vi "Centauro Verify LED Scroll.vi"(8 "Error In":errorcluster, 10 "#Retries":i32=20, 11 "GEA2 Reference In":refnum<k24>) -> (0 "Error Out":errorcluster, 2 "Pass/Fail?":bool, 3 "GEA2 Reference Out":refnum<k24>)   [LabVIEW 2016]
uses:
  Q:/Common/DLLs/GEA3/GeaCommunication.dll
  Common/DLLs/GEA3/GeaCommunication.dll
  Centauro Washer/Product Testcode/Centauro/Valew Common/type defs/LED Status OOB.ctl
  Common/LabVIEW GEA2 Toolkit/LabVIEW_GEA2_Toolkit.lvlibp
panel:
  in  "Board Index":i32
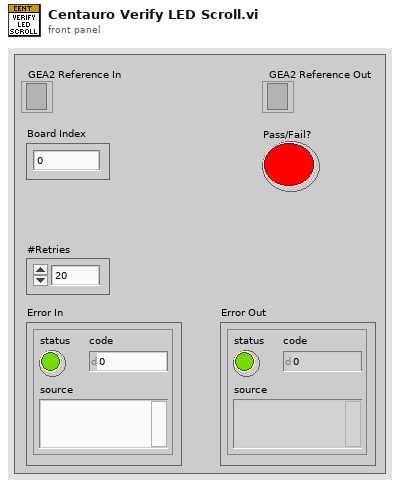
[diagram p1: front panel]
types:
  T1 = typedef "LED Status OOB.ctl" = enum32{"Off", "On", "Blink"}
  T2 = cluster{"Damp":T1, "Dry":T1, "Cool":T1, "Eco":T1}
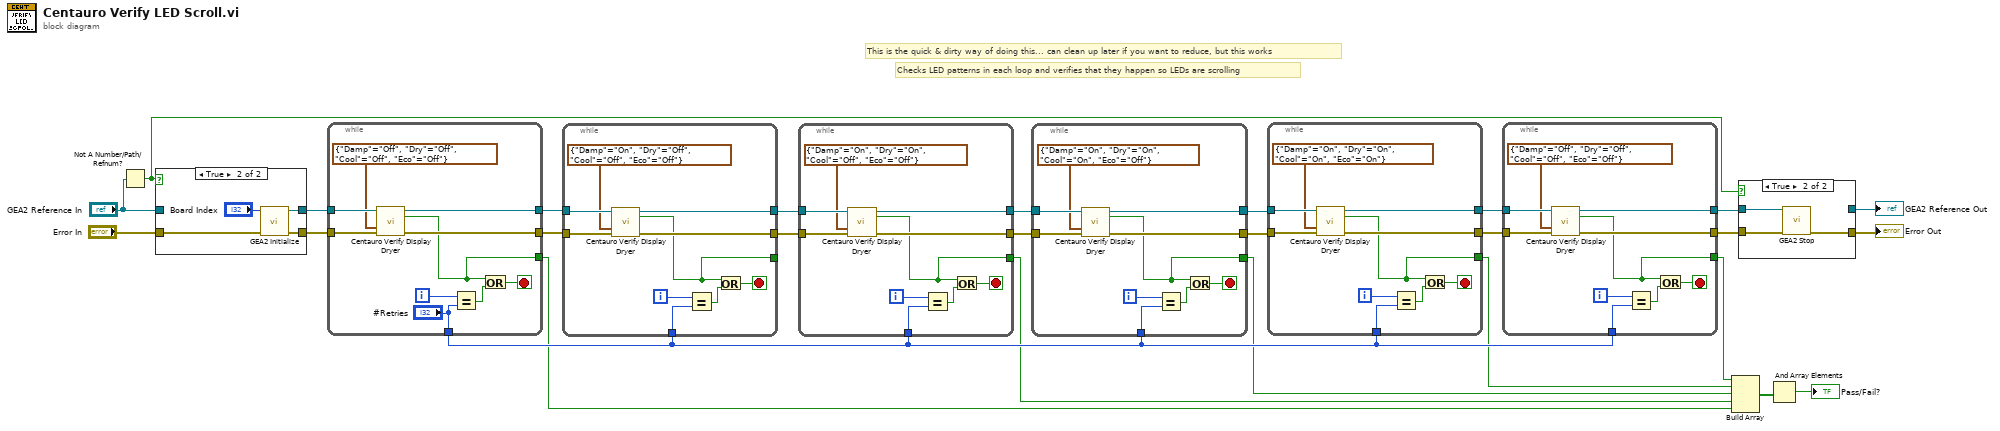
[diagram p0: block diagram]
diagram:
  # "Checks LED patterns in each loop and verifies that they happen so LEDs are scrolling"
  # "This is the quick & dirty way of doing this... can clean up later if you want to reduce, but this works"
  n1 = Not A Number/Path/Refnum?(number/path/refnum="GEA2 Reference In") -> (NaN/Path/Refnum?=w2:bool)
  n2 = case shown="True" w2 {
    tunnel: [w28 w33] -> w25
    tunnel: "Error In" -> [w28 w32]
    tunnel: [w29 w31] -> w26
    tunnel: "GEA2 Reference In" -> [w29 _]
    frame False {
    }
    frame True {
      n3 = call "GEA2 Initialize.vi"("Board Index"="Board Index", "error in"=w32) -> ("GEA2 Reference Out"=w31:refnum<k24>, "error out"=w33:errorcluster)  [unwired: 11 in, 1 out]
    }
  }
  n4 = while {
    tunnel: w26 -> [w43]
    tunnel: w25 -> [w42]
    tunnel: [w41] -> w24
    tunnel: [w40] -> w23
    tunnel: [w37] -> w9
    tunnel: ["#Retries"] -> w14
    i -> [w36]
    stop <- w38 stop-if-true
    n5 = call "Centauro Verify Display Dryer.vi"("GEA2 Reference In"=w43, "Expected LED Status"=T2 {"Damp"=enum."Off", "Dry"=enum."Off", "Cool"=enum."Off", "Eco"=enum."Off"}, "Error In"=w42) -> ("GEA2 Reference Out"=w41:refnum<k24>, "Pass/Fail?"=w37:bool, "Error Out"=w40:errorcluster)  [unwired: 7 in, 3 out]
    n6 = Equal?(x=w36, y="#Retries") -> (x = y?=w39:bool)
    n7 = Or(x=w37, y=w39) -> (x .or. y?=w38:bool)
  }
  n8 = while {
    tunnel: w24 -> [w53]
    tunnel: w23 -> [w52]
    tunnel: [w51] -> w22
    tunnel: [w50] -> w21
    tunnel: [w47] -> _
    tunnel: w14 -> [w45]
    i -> [w46]
    stop <- w48 stop-if-true
    n9 = call "Centauro Verify Display Dryer.vi"("GEA2 Reference In"=w53, "Expected LED Status"=T2 {"Damp"=enum."On", "Dry"=enum."Off", "Cool"=enum."Off", "Eco"=enum."Off"}, "Error In"=w52) -> ("GEA2 Reference Out"=w51:refnum<k24>, "Pass/Fail?"=w47:bool, "Error Out"=w50:errorcluster)  [unwired: 7 in, 3 out]
    n10 = Equal?(x=w46, y=w45) -> (x = y?=w49:bool)
    n11 = Or(x=w47, y=w49) -> (x .or. y?=w48:bool)
  }
  n12 = while {
    tunnel: w22 -> [w63]
    tunnel: w21 -> [w62]
    tunnel: [w61] -> w20
    tunnel: [w60] -> w19
    tunnel: [w57] -> w10
    tunnel: w14 -> [w55]
    i -> [w56]
    stop <- w58 stop-if-true
    n13 = call "Centauro Verify Display Dryer.vi"("GEA2 Reference In"=w63, "Expected LED Status"=T2 {"Damp"=enum."On", "Dry"=enum."On", "Cool"=enum."Off", "Eco"=enum."Off"}, "Error In"=w62) -> ("GEA2 Reference Out"=w61:refnum<k24>, "Pass/Fail?"=w57:bool, "Error Out"=w60:errorcluster)  [unwired: 7 in, 3 out]
    n14 = Equal?(x=w56, y=w55) -> (x = y?=w59:bool)
    n15 = Or(x=w57, y=w59) -> (x .or. y?=w58:bool)
  }
  n16 = while {
    tunnel: w20 -> [w73]
    tunnel: w19 -> [w72]
    tunnel: [w71] -> w18
    tunnel: [w70] -> w17
    tunnel: [w67] -> w11
    tunnel: w14 -> [w65]
    i -> [w66]
    stop <- w68 stop-if-true
    n17 = call "Centauro Verify Display Dryer.vi"("GEA2 Reference In"=w73, "Expected LED Status"=T2 {"Damp"=enum."On", "Dry"=enum."On", "Cool"=enum."On", "Eco"=enum."Off"}, "Error In"=w72) -> ("GEA2 Reference Out"=w71:refnum<k24>, "Pass/Fail?"=w67:bool, "Error Out"=w70:errorcluster)  [unwired: 7 in, 3 out]
    n18 = Equal?(x=w66, y=w65) -> (x = y?=w69:bool)
    n19 = Or(x=w67, y=w69) -> (x .or. y?=w68:bool)
  }
  n20 = while {
    tunnel: w18 -> [w83]
    tunnel: w17 -> [w82]
    tunnel: [w81] -> w16
    tunnel: [w80] -> w15
    tunnel: [w77] -> w12
    tunnel: w14 -> [w75]
    i -> [w76]
    stop <- w78 stop-if-true
    n21 = call "Centauro Verify Display Dryer.vi"("GEA2 Reference In"=w83, "Expected LED Status"=T2 {"Damp"=enum."On", "Dry"=enum."On", "Cool"=enum."On", "Eco"=enum."On"}, "Error In"=w82) -> ("GEA2 Reference Out"=w81:refnum<k24>, "Pass/Fail?"=w77:bool, "Error Out"=w80:errorcluster)  [unwired: 7 in, 3 out]
    n22 = Equal?(x=w76, y=w75) -> (x = y?=w79:bool)
    n23 = Or(x=w77, y=w79) -> (x .or. y?=w78:bool)
  }
  n24 = while {
    tunnel: w16 -> [w93]
    tunnel: w15 -> [w92]
    tunnel: [w91] -> w3
    tunnel: [w90] -> w4
    tunnel: [w87] -> w13
    tunnel: w14 -> [w85]
    i -> [w86]
    stop <- w88 stop-if-true
    n25 = call "Centauro Verify Display Dryer.vi"("GEA2 Reference In"=w93, "Expected LED Status"=T2 {"Damp"=enum."Off", "Dry"=enum."Off", "Cool"=enum."Off", "Eco"=enum."Off"}, "Error In"=w92) -> ("GEA2 Reference Out"=w91:refnum<k24>, "Pass/Fail?"=w87:bool, "Error Out"=w90:errorcluster)  [unwired: 7 in, 3 out]
    n26 = Equal?(x=w86, y=w85) -> (x = y?=w89:bool)
    n27 = Or(x=w87, y=w89) -> (x .or. y?=w88:bool)
  }
  n28 = Build Array(w13, w12, w11, w10, w9) -> (w8:bool[])
  n29 = case shown="True" w2 {
    tunnel: [w94 w98] -> w6
    tunnel: [w95 _] -> w5
    tunnel: w3 -> [w95 w97]
    tunnel: w4 -> [w94 w96]
    frame False {
    }
    frame True {
      n30 = call "GEA2 Stop.vi"("GEA2 Reference In"=w97, "Error In"=w96) -> ("Error Out"=w98:errorcluster)  [unwired: 13 in]
    }
  }
  "GEA2 Reference Out" <- w5
  "Error Out" <- w6
  n31 = And Array Elements(Boolean array=w8) -> (logical AND=→"Pass/Fail?":bool)
